vi "Example2.vi"() -> ()   [LabVIEW 2020]
doc: "Simple example of file operations with error handling. Comments in polish language."
uses:
  <vilib>/Utility/file.llb/Write Delimited Spreadsheet (DBL).vi
  <vilib>/Utility/file.llb/Read Delimited Spreadsheet (DBL).vi
panel:
  in  "Load":bool
  in  "Clear":bool
  out "Graph":dbl[](graph) caption="Obecny pomiar"
  in  "GetData":bool
  in  "SaveData":bool
  in  "stop":bool
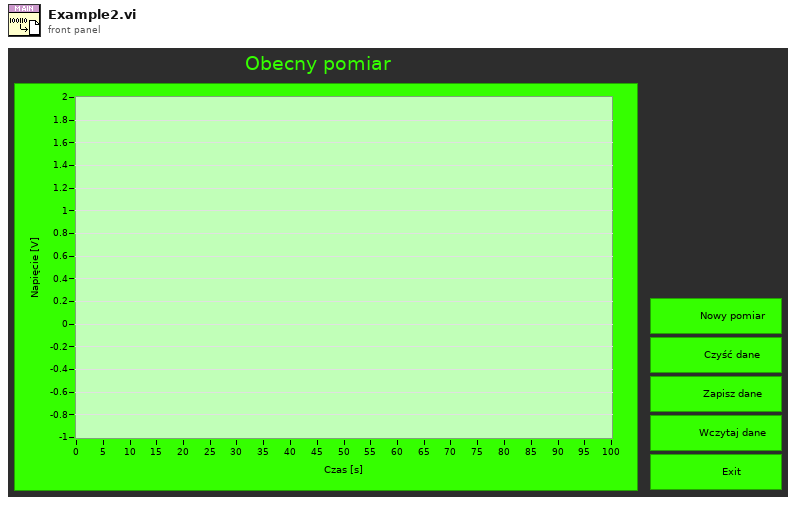
[diagram p1: front panel]
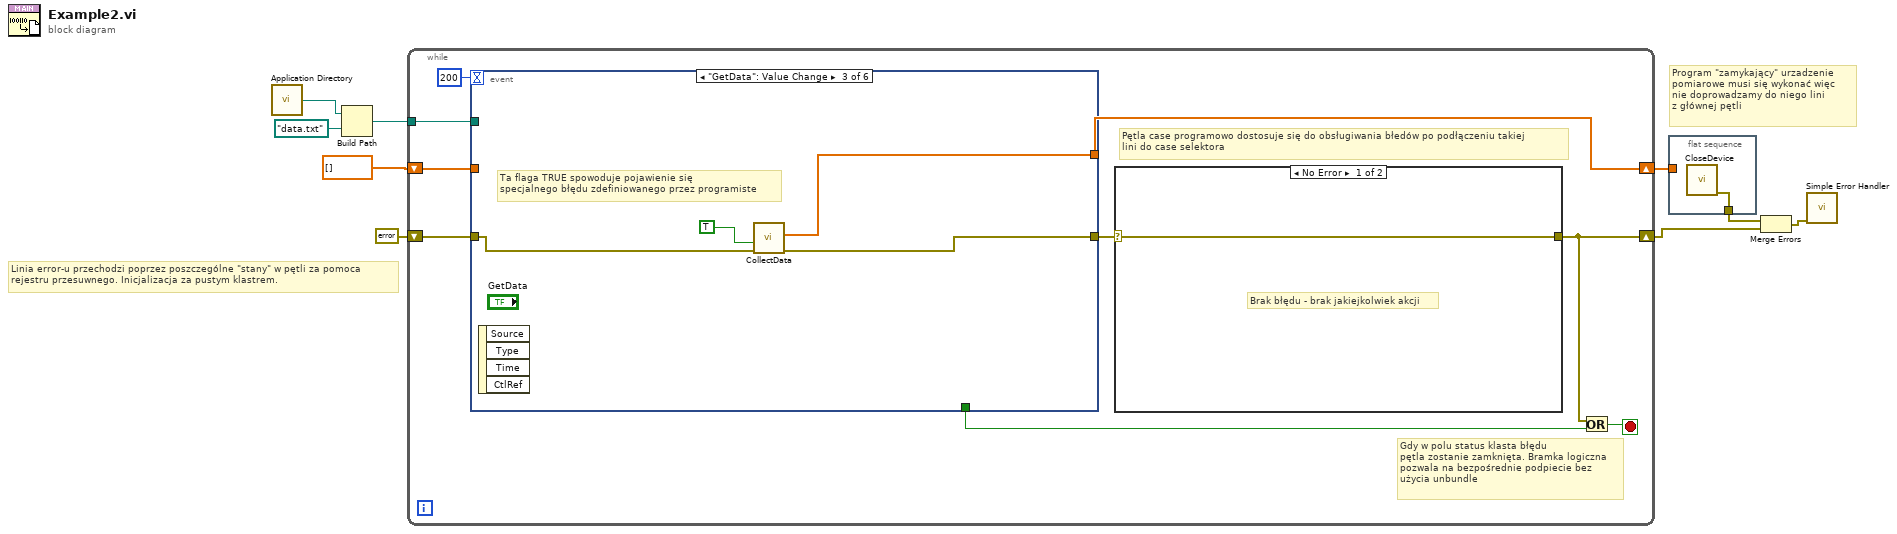
[diagram p0: block diagram]
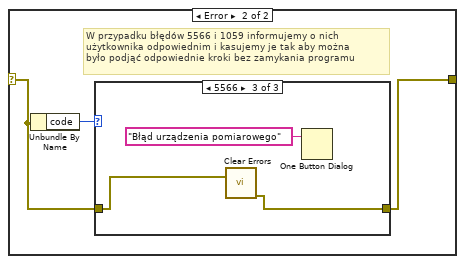
[diagram p2: hidden frame]
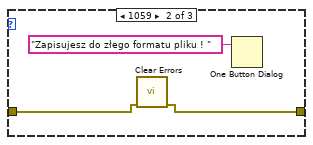
[diagram p4: hidden frame]
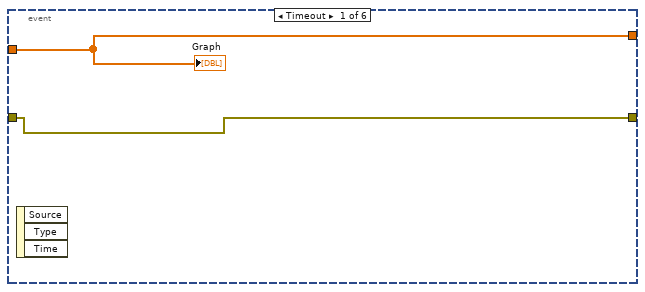
[diagram p5: hidden frame]
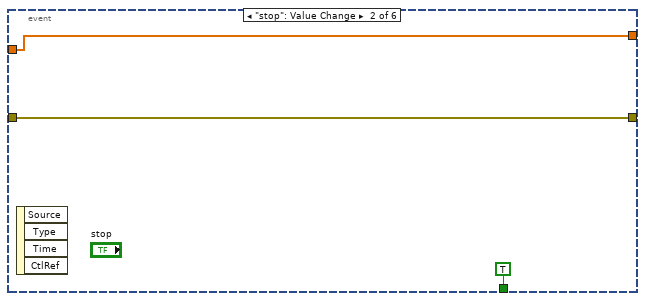
[diagram p6: hidden frame]
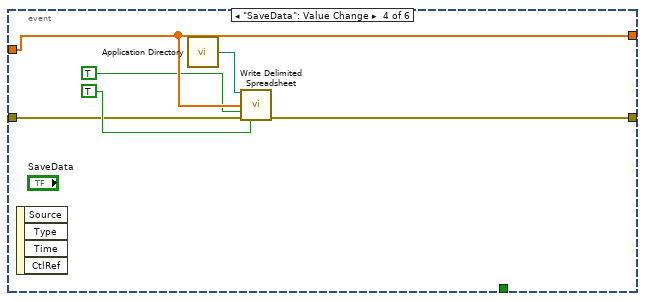
[diagram p7: hidden frame]
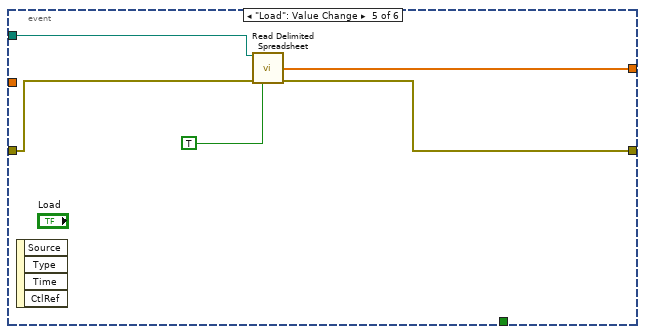
[diagram p8: hidden frame]
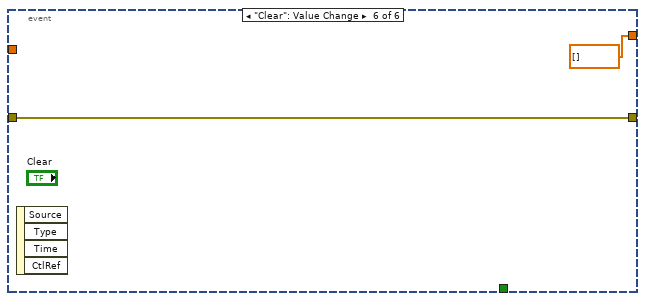
[diagram p9: hidden frame]
diagram:
  # "Program \"zamykający\" urzadzenie\npomiarowe musi się wykonać więc\nnie doprowadzamy do niego lini\nz głównej pętli"
  # "Linia error-u przechodzi poprzez poszczególne \"stany\" w pętli za pomoca \nrejestru przesuwnego. Inicjalizacja za pustym klastrem."
  n1 = call <vilib>:"Application Directory.vi"() -> ("Application Directory"=w7:path)
  n2 = Build Path(base path=w7, name or relative path=path "data.txt") -> (appended path=w6:path)
  n3 = while {
    shift-right: [w16] -> w1
    shift-left: dbl[] [] -> [w17]
    tunnel: w6 -> [w14]
    shift-right: [w10] -> w2
    shift-left: errorcluster {"status"=FALSE, "code"=0, "source"=""} ("error out") -> [w13]
    stop <- w12 stop-if-true
    # "Pętla case programowo dostosuje się do obsługiwania błedów po podłączeniu takiej \nlini do case selektora"
    # "Gdy w polu status klasta błędu \npętla zostanie zamknięta. Bramka logiczna\npozwala na bezpośrednie podpiecie bez \nużycia unbundle"
    n4 = event shown="[2] \"GetData\": Value Change" {
      selector: _ -> [_ _ _ _ _ _]
      dyn-events: _ -> [_ _ _ _ _ _]
      timeout: 200 -> [_ _ _ _ _ _]
      tunnel: w17 -> [w31 w33 _ w44 _ _]
      tunnel: [w31 w33 w38 w44 w49 dbl[] [] ("Data")] -> w16
      tunnel: [_ TRUE ("stop") _ _ _ _] -> w15
      tunnel: w14 -> [_ _ _ _ w48 _]
      tunnel: [w30 w32 w36 w41 w45 w50] -> w11
      tunnel: w13 -> [w30 w32 w37 w40 w46 w50]
      event Timeout {
        n5 = event-data() -> ()  [unwired: 1 in, 3 out]
        "Graph" <- w31
      }
      event "stop": Value Change {
        n6 = event-data() -> ()  [unwired: 1 in, 4 out]
      }
      event "GetData": Value Change {
        # "Ta flaga TRUE spowoduje pojawienie się \nspecjalnego błędu zdefiniowanego przez programiste"
        n7 = event-data() -> ()  [unwired: 1 in, 4 out]
        n8 = call "CollectData.vi"("Error In"=w37, "SimErr"=TRUE) -> ("Error Out"=w36:errorcluster, "Data"=w38:dbl[])  [unwired: 4 in]
      }
      event "SaveData": Value Change {
        n9 = event-data() -> ()  [unwired: 1 in, 4 out]
        n10 = call <vilib>:"Application Directory.vi"() -> ("Application Directory"=w39:path)
        n11 = call-poly <vilib>:"Write Delimited Spreadsheet.vi"("file path (dialog if empty)"=w39, "1D data"=w44, "append to file? (new file:F)"=TRUE, "error in (no error)"=w40, "transpose? (no:F)"=TRUE) -> ("error out"=w41:errorcluster)  [unwired: 9 in, 1 out]
      }
      event "Load": Value Change {
        n12 = event-data() -> ()  [unwired: 1 in, 4 out]
        n13 = call-poly <vilib>:"Read Delimited Spreadsheet.vi"("file path (dialog if empty)"=w48, "error in (no error)"=w46, "transpose? (F)"=TRUE) -> ("first row"=w49:dbl[], "error out"=w45:errorcluster)  [unwired: 7 in, 4 out]
      }
      event "Clear": Value Change {
        n14 = event-data() -> ()  [unwired: 1 in, 4 out]
      }
    }
    n15 = case shown="No Error" w11 {
      selector: w11 -> [w19 w21]
      tunnel: [w19 w20] -> w10
      frame No Error {
        # "Brak błędu - brak jakiejkolwiek akcji"
      }
      frame Error {
        # "W przypadku błędów 5566 i 1059 informujemy o nich\nużytkownika odpowiednim i kasujemy je tak aby można\nbyło podjąć odpowiednie kroki bez zamykania programu"
        n16 = Unbundle By Name(w21) -> ("code"=w22:i32)
        n17 = case shown="5566" w22 {
          tunnel: w21 -> [w23 w25 w28]
          tunnel: [w23 w24 w27] -> w20
          frame 0, Default {
            # "W tym przypadku pozwalamy na dalsza \npropagacje aby zamknąc program"
          }
          frame 1059 {
            n18 = call <vilib>:"Clear Errors.vi"("error in (no error)"=w25) -> ("error out"=w24:errorcluster)  [unwired: 5 in, 1 out]
            n19 = One Button Dialog(message="Zapisujesz do złego formatu pliku ! ") -> ()  [unwired: 1 in, 1 out]
          }
          frame 5566 {
            n20 = call <vilib>:"Clear Errors.vi"("error in (no error)"=w28) -> ("error out"=w27:errorcluster)  [unwired: 5 in, 1 out]
            n21 = One Button Dialog(message="Błąd urządzenia pomiarowego") -> ()  [unwired: 1 in, 1 out]
          }
        }
      }
    }
    n22 = Or(x=w10, y=w15) -> (x .or. y?=w12:bool)
  }
  n23 = flat-sequence {
    tunnel: [w52] -> w4
    tunnel: w1 -> [_]
    frame #0 {
      n24 = call "CloseDevice.vi"() -> ("Error Out"=w52:errorcluster)  [unwired: 7 in]
    }
  }
  n25 = Merge Errors(w4, w2) -> (w3:errorcluster)
  n26 = call <vilib>:"Simple Error Handler.vi"("error in (no error)"=w3) -> ()  [unwired: 4 in, 5 out]
